vi "Test HTTP Response.vi"() -> ()   [LabVIEW 2023, in "VolatusSeq.lvlib" / "State.lvclass"]
uses:
  State.lvclass
  <vilib>/httpClient/LabVIEWHTTPClient.lvlib
panel:
  out "error out":errorcluster
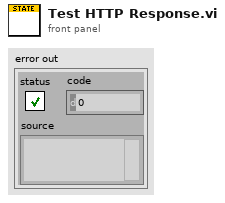
[diagram p1: front panel]
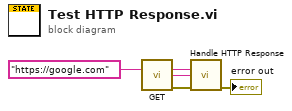
[diagram p0: block diagram]
diagram:
  n1 = call <vilib>:"GET.vi"("url"="https://google.com") -> ("headers"=w3:string, "body"=w4:string, "error out"=w5:errorcluster)  [unwired: 11 in, 1 out]
  n2 = call "Handle HTTP Response.vi"("Headers"=w3, "Body"=w4, "error in (no error)"=w5) -> ("error out"=→"error out":errorcluster)  [unwired: 12 in]
